vi "Data Trends.vi"(8 "error in (no error)":errorcluster, 9 "Hours":dbl=4000.0 format="%#_13g", 10 "Sample":dbl=21.0 format="%#_13g", 11 "Model":dbl=5.0 format="%#_13g") -> (0 "error out":errorcluster, 1 "Percent Flicker":T1={"XY Graph 2"=[{[{0.0, "Numeric"=0.97}, {1000.0, "Numeric"=0.9733}, {2000.0, "Numeric"=0.97}, {3000.0, "Numeric"=0.97}]}, {[{4000.0, "Numeric"=0.97346}]}, {[{0.0, "Numeric"=0.9713197181503324}, {1000.0, "Numeric"=0.970989831390721}, {2000.0, "Numeric"=0.9706600566696818}, {3000.0, "Numeric"=0.9703303939491632}, {4000.0, "Numeric"=0.9700008431911267}]}, {[{0.0, "Numeric"=0.9822728418829588}, {1000.0, "Numeric"=0.9805677813713304}, {2000.0, "Numeric"=0.9802376627629179}, {3000.0, "Numeric"=0.9812824860577213}, {4000.0, "Numeric"=0.9837022512557407}]}, {[{0.0, "Numeric"=0.9603665944139}, {1000.0, "Numeric"=0.9614118814215039}, {2000.0, "Numeric"=0.9610824505649396}, {3000.0, "Numeric"=0.9593783018442069}, {4000.0, "Numeric"=0.9562994352593058}]}], "Out of Range"=FALSE}, 2 "Power Factor":T1={"XY Graph 2"=[{[{0.0, "Numeric"=0.97}, {1000.0, "Numeric"=0.9733}, {2000.0, "Numeric"=0.97}, {3000.0, "Numeric"=0.97}]}, {[{4000.0, "Numeric"=0.97346}]}, {[{0.0, "Numeric"=0.9713197181503324}, {1000.0, "Numeric"=0.970989831390721}, {2000.0, "Numeric"=0.9706600566696818}, {3000.0, "Numeric"=0.9703303939491632}, {4000.0, "Numeric"=0.9700008431911267}]}, {[{0.0, "Numeric"=0.9822728418829588}, {1000.0, "Numeric"=0.9805677813713304}, {2000.0, "Numeric"=0.9802376627629179}, {3000.0, "Numeric"=0.9812824860577213}, {4000.0, "Numeric"=0.9837022512557407}]}, {[{0.0, "Numeric"=0.9603665944139}, {1000.0, "Numeric"=0.9614118814215039}, {2000.0, "Numeric"=0.9610824505649396}, {3000.0, "Numeric"=0.9593783018442069}, {4000.0, "Numeric"=0.9562994352593058}]}], "Out of Range"=FALSE}, 3 "Power":T1={"XY Graph 2"=[{[{0.0, "Numeric"=0.97}, {1000.0, "Numeric"=0.9733}, {2000.0, "Numeric"=0.97}, {3000.0, "Numeric"=0.97}]}, {[{4000.0, "Numeric"=0.97346}]}, {[{0.0, "Numeric"=0.9713197181503324}, {1000.0, "Numeric"=0.970989831390721}, {2000.0, "Numeric"=0.9706600566696818}, {3000.0, "Numeric"=0.9703303939491632}, {4000.0, "Numeric"=0.9700008431911267}]}, {[{0.0, "Numeric"=0.9822728418829588}, {1000.0, "Numeric"=0.9805677813713304}, {2000.0, "Numeric"=0.9802376627629179}, {3000.0, "Numeric"=0.9812824860577213}, {4000.0, "Numeric"=0.9837022512557407}]}, {[{0.0, "Numeric"=0.9603665944139}, {1000.0, "Numeric"=0.9614118814215039}, {2000.0, "Numeric"=0.9610824505649396}, {3000.0, "Numeric"=0.9593783018442069}, {4000.0, "Numeric"=0.9562994352593058}]}], "Out of Range"=FALSE}, 4 "Keep Data":bool)   [LabVIEW 2014, in "Data Trends.lvlib"]
uses:
  Data Trends.lvlib
  Check New Data Point.ctl
  <vilib>/Analysis/1siggen.llb/Ramp Pattern by Delta.vi
  <vilib>/Analysis/NI_AALBase.lvlib
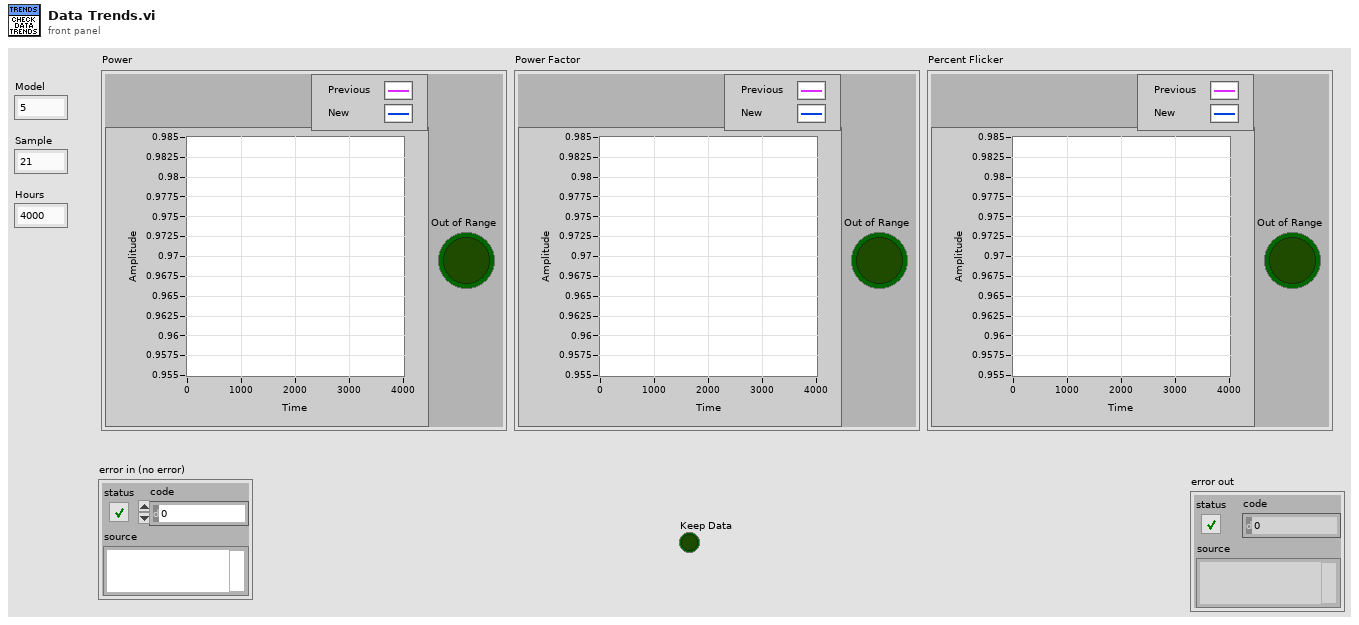
[diagram p1: front panel]
types:
  T1 = typedef "Data Trends.lvlib/Check New Data Point.ctl" = cluster{"XY Graph 2":cluster{cluster{dbl, "Numeric":dbl}[]}[], "Out of Range":bool}
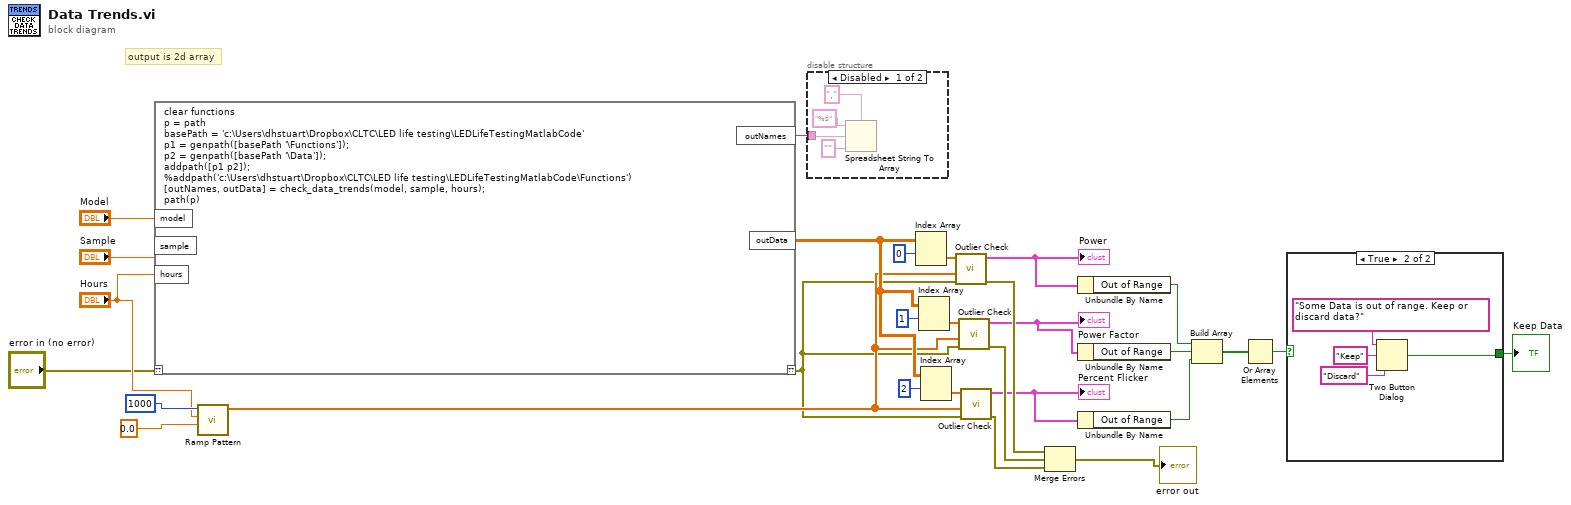
[diagram p0: block diagram]
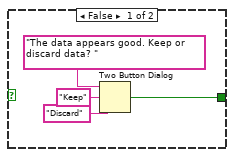
[diagram p3: hidden frame]
diagram:
  # "output is 2d array"
  n1 = script code="clear functions\np = path\nbasePath = 'c:\\Users\\dhstuart\\Dropbox\\CLTC\\LED life testing\\LEDLifeTestingMatlabCode'\np1 = genpath([basePath '\\Functions']);\np2 = genpath([basePath '\\Data']);\naddpath([p1 p2]);\n%addpath('c:\\Users\\dhstuart\\Dropbox\\CLTC\\LED life testing\\LEDLifeTestingMatlabCode\\Functions')\n[outNames, outData] = check_data_trends(model, sample, hours);\npath(p)"("??"="error in (no error)", "model"="Model", "sample"="Sample", "hours"="Hours") -> ("??"=w18:errorcluster, "outNames"=w24:string, "outData"=w23:dbl[][])
  n2 = call-poly <vilib>:"Ramp Pattern.vi"("start"=0.0, "end"="Hours", "delta"=1000 ("samples")) -> ("Ramp Pattern"=w22:dbl[])  [unwired: 6 in, 2 out]
  n3 = disable-structure shown="Disabled" {
    disable-tunnel: w24 -> [w33 _]
    frame Disabled {
      n4 = Spreadsheet String To Array(delimiter (Tab)=",", format string="%s", spreadsheet string=w33, array type (2D Dbl)="" ("delimiter (Tab)")) -> ()  [unwired: 1 out]
    }
    frame Enabled {
    }
  }
  n5 = Index Array(array=w23, index (row)=0) -> (element=w14:dbl[])  [unwired: 1 in]
  n6 = Index Array(array=w23, index (row)=1) -> (element=w13:dbl[])  [unwired: 1 in]
  n7 = Index Array(array=w23, index (row)=2) -> (element=w16:dbl[])  [unwired: 1 in]
  n8 = call "Outlier Check.vi"("error in (no error)"=w18, "New Hours"=w22, "New Data"=w14) -> ("error out"=w21:errorcluster, "Check New Data Point 2"=w10:T1)  [unwired: 7 in]
  "Power" <- w10
  n9 = call "Outlier Check.vi"("error in (no error)"=w18, "New Hours"=w22, "New Data"=w13) -> ("error out"=w20:errorcluster, "Check New Data Point 2"=w9:T1)  [unwired: 7 in]
  "Power Factor" <- w9
  n10 = call "Outlier Check.vi"("error in (no error)"=w18, "New Hours"=w22, "New Data"=w16) -> ("error out"=w19:errorcluster, "Check New Data Point 2"=w8:T1)  [unwired: 7 in]
  "Percent Flicker" <- w8
  n11 = Merge Errors(w21, w20, w19) -> (→"error out":errorcluster)
  n12 = Unbundle By Name(w10) -> ("Out of Range"=w7:bool)
  n13 = Unbundle By Name(w9) -> ("Out of Range"=w6:bool)
  n14 = Unbundle By Name(w8) -> ("Out of Range"=w5:bool)
  n15 = Build Array(w7, w6, w5) -> (w4:bool[])
  n16 = Or Array Elements(Boolean array=w4) -> (logical OR=w3:bool)
  n17 = case shown="True" w3 {
    tunnel: [w34 w38] -> w2
    frame False {
      n18 = Two Button Dialog(message="The data appears good. Keep or discard data? ", 1:"Discard" ("F button name (\"Cancel\")"), 2:"Keep" ("T button name (\"OK\")")) -> (T button?=w34:bool)
    }
    frame True {
      n19 = Two Button Dialog(message="Some Data is out of range. Keep or discard data?", 1:"Discard" ("F button name (\"Cancel\")"), 2:"Keep" ("T button name (\"OK\")")) -> (T button?=w38:bool)
    }
  }
  "Keep Data" <- w2
